vi "cmd_open_form.vi"(8 "error in (no error)":errorcluster, 11 "JSON":string) -> (0 "error out":errorcluster)   [LabVIEW 2021]
doc: "Opens the GUI window specified in the argument\n\n :param name: Specifies the form name"
panel:
  out "args":cluster{"name":string}
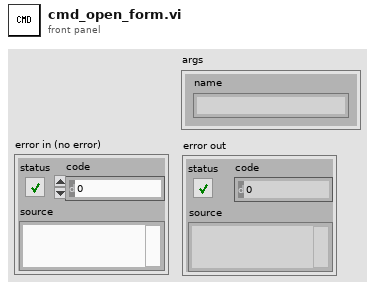
[diagram p1: front panel]
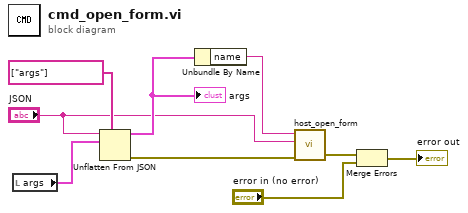
[diagram p0: block diagram]
diagram:
  n1 = local read "args"() -> (w8:cluster{"name":string})
  n2 = Unflatten From JSON(path=string[] ["args"], JSON string="JSON", type and defaults=w8) -> (value=w7:cluster{"name":string}, error out=w6:errorcluster)  [unwired: 4 in]
  "args" <- w7
  n3 = Unbundle By Name(w7) -> ("name"=w2:string)
  n4 = call "host_open_form.vi"("error in (no error)"=w6, "JSON"="JSON", "name"=w2) -> ("error out"=w5:errorcluster)  [unwired: 8 in]
  n5 = Merge Errors(w5, "error in (no error)") -> (→"error out":errorcluster)
